vi "sendValue.vi"(8 "error in (no error)":errorcluster, 10 "data":variant, 11 "moveAzimuth in":refnum<class "moveAzimuth.lvclass">) -> (0 "error out":errorcluster, 2 "function return":i32, 3 "moveAzimuth out":refnum<class "moveAzimuth.lvclass">)   [LabVIEW 2016, in "SALLV_AtDome_Messaging.lvlib" / "moveAzimuth.lvclass"]
uses:
  moveAzimuth.lvclass
  ts_sallv_AtDome/DataTypes/command_moveAzimuth.ctl
  ts_sallv_AtDome/SALLV_AtDome.lvlib
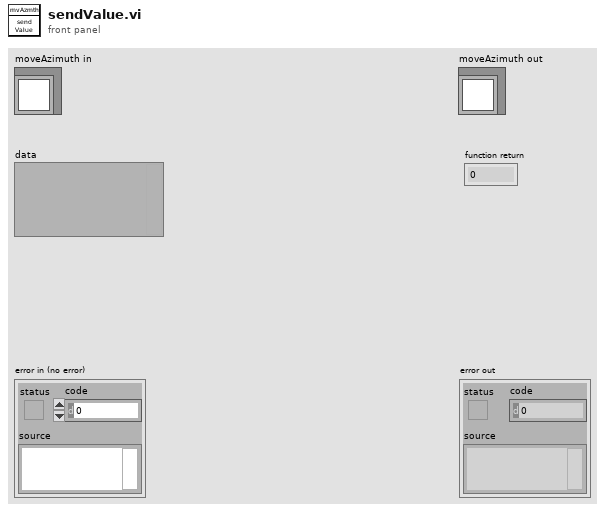
[diagram p1: front panel]
types:
  T1 = typedef "SALLV_AtDome.lvlib/command_moveAzimuth.ctl" = cluster{"azimuth":sgl}
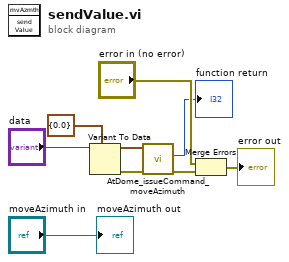
[diagram p0: block diagram]
diagram:
  n1 = Variant To Data(type=T1 {"azimuth"=0.0} ("data"), Variant="data") -> (data=w3:T1, error out=w5:errorcluster)  [unwired: 1 in]
  n2 = call "AtDome_issueCommand_moveAzimuth.vi"("error in (no error)"=w5, "command_moveAzimuth_Ctl"=w3) -> ("error out"=w1:errorcluster, "function return"=→"function return":i32)  [unwired: 7 in, 1 out]
  n3 = Merge Errors("error in (no error)", w1) -> (→"error out":errorcluster)
  "moveAzimuth out" <- "moveAzimuth in"
